vi "Com _Change.vi"(7 "NewPSW":string, 8 "error in (no error)":errorcluster caption="错误输入（无错误）", 9 "OldPSW":string, 10 "UserNo":string, 11 "Traceability 引用句柄":refnum<k24>) -> (0 "error out":errorcluster caption="错误输出", 2 "Com_ChangePSW":string, 3 "Traceability 引用句柄输出":refnum<k24>)   [LabVIEW 2014, in "Traceability.lvlib"]
uses:
  D:/webservice/Traceability.dll
  Traceability.dll
  Traceability.lvlib
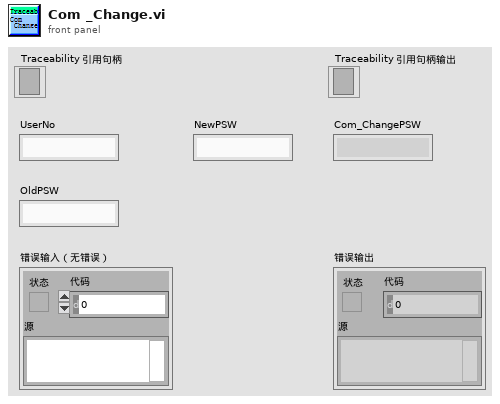
[diagram p1: front panel]
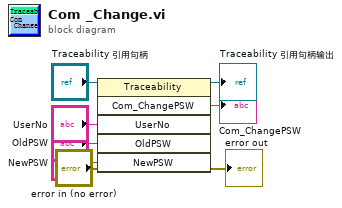
[diagram p0: block diagram]
diagram:
  n1 = invoke class="Traceability" method="Com_ChangePSW"(reference="Traceability 引用句柄", error in="error in (no error)", "UserNo"="UserNo", "OldPSW"="OldPSW", "NewPSW"="NewPSW") -> (reference out=→"Traceability 引用句柄输出":refnum<k24>, error out=→"error out":errorcluster, "Com_ChangePSW"=→"Com_ChangePSW":string)  [unwired: 1 in, 3 out]
